vi "AlliGator Computer IRF t_0 and Mean Lifetime.vi"(8 "error in":errorcluster, 11 "Reference Decay":cluster{"t Array":dbl[], "I Array":dbl[]}) -> (0 "error out":errorcluster, 1 "t_0":dbl, 2 "<tau>_IRF":dbl)   [LabVIEW 2021, in "AlliGator Decay Processing.lvlib"]
doc: "Computes an estimate of the average lifetime of the IRF and the location of the rising time."
uses:
  AlliGator Decay Processing.lvlib
  Settings/AlliGator Settings List.ctl
  Settings/AlliGator Average Lifetime Options.ctl
  Graphs/XY Graph/XY Graph Add-Ons.lvlib
  Settings/AlliGator Settings.lvlib
  IRF/AlliGator IRF.lvlib
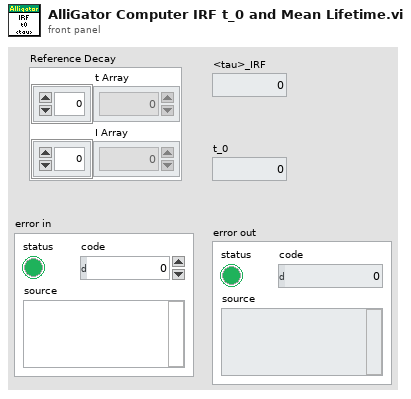
[diagram p1: front panel]
types:
  T1 = typedef "AlliGator Settings.lvlib/AlliGator Average Lifetime Options.ctl" = cluster{"Use Local IRF ":bool, "Use IRF Offset":bool, "Use Fixed Offset":bool, "Fixed Offset":dbl[unit], "Baseline %":dbl}
  T2 = typedef "AlliGator Settings.lvlib/AlliGator Settings List.ctl" = enum16{"GUI:Visible Settings Tab", "GUI:Last Run Version", "Source Image:Use Image Histogram for Contrast", "Source Image:Low Count Pixels Rejection Options", "Source Image:High Count Pixels Rejection Options", "Source Image:Use Image Brightness", "Source Image:Blend Overlay with Image Background", "Source Image:Use Fixed ROI Diameter", "Source Image:ROI Diameter", "Source Image:ROI Center Color", "Source Image:Peak Threshold", "Source Image:Intensity Threshold", "Source Image:Image Binning Options", "Source Image:Image Smoothing Options", "Source Image:Image Histogram Active", "Source Image:Invert Binary Mask", "Source Image:Hot Pixel Removal", "Source Image:Overlay Analyzed ROI Center", "Source Image:Auto-Adjust Contrast", "Source Image:Histogram Lower Percentile", "Source Image:Histogram Upper Percentile", "Source Image:Save Source Image", "Source Image:Scale Bar Options", "Source Image:Image Resolution (Pixel Size)", "Source Image:Flatfield Correction", "Source Image:Show Dead Left Columns Correction", "Source Image:Dead Left Columns Correction", "Source Image:Image Pre-Processing Operations Order", "Source Image:Overlay ROI Median", "Source Image:Median Overlay Color", "Data Information:Gate Width", "Data Information:Nanotime Gate Separation", "Data Information:Macrotime Gate Separation", "Data Information:Gate Step", "Data Information:# Gates", "Data Information:Gate Image Exposure", "Data Information:Gate Image Integration", "Data Information:Gates to Skip", "Data Information:Gates to Keep", "Data Information:Define Gates to", "Data Information:Channel Name", "Data Information:Available Channel Names", "Data Information:Channel Arithmetic", "Data Information:Background File Subtraction", "Data Information:Background File", "Data Information:Background Scaling Factor", "Data Information:Background Pile-up Correction", "Data Information:Background Pixel Well Capacity", "Data Information:Laser Period", "Data Information:SYNC Period", "Data Information:Pile-up Correction", "Data Information:Pixel Well Capacity", "Data Information:Dataset Scaling Factor", "Fluorescence Decay_Decay Pre-Processing:Reverse Gates", "Fluorescence Decay_Decay Pre-Processing:Verbose Decay Pre-Processing", "Fluorescence Decay_Decay Pre-Processing:Use Decay Pre-Processing", "Fluorescence Decay_Decay Pre-Processing:Background Subtraction", "Fluorescence Decay_Decay Pre-Processing:Background Definition Range", "Fluorescence Decay_Decay Pre-Processing:Baseline Subtraction Method", "Fluorescence Decay_Decay Pre-Processing:Decay Pre-Processing Operations Order", "Fluorescence Decay_Decay Pre-Processing:Smoothing Parameter", "Fluorescence Decay_Decay Pre-Processing:Shift Decay", "Fluorescence Decay_Decay Pre-Processing:Decay Shift Parameters", "Fluorescence Decay_Decay Pre-Processing:Fold Decay", "Fluorescence Decay_Decay Pre-Processing:# Folds", "Fluorescence Decay_Decay Pre-Processing:1-Normalize Decay", "Fluorescence Decay_Decay Pre-Processing:[0-1]-Normalize Decay", "Fluorescence Decay_Decay Pre-Processing:Smoothen Decay", "Fluorescence Decay_Decay Pre-Processing:Extrapolate Decay", "Fluorescence Decay_Decay Pre-Processing:Use Periodicity", "Fluorescence Decay_Decay Pre-Processing:Use Cursors", "Fluorescence Decay_Decay Pre-Processing:Tail Fraction", "Fluorescence Decay_Decay Pre-Processing:Head Fraction", "Fluorescence Decay_Decay Pre-Processing:Additional Points", "Fluorescence Decay_Decay Pre-Processing:Straighten Decay", "Fluorescence Decay_Decay Pre-Processing:Constant Background", "Fluorescence Decay_Decay Pre-Processing:Pixel-Normalize Decay", "Fluorescence Decay_Advanced Analysis:Extract IRF instead of Decay", "Fluorescence Decay_Advanced Analysis:IRF Extraction Options", "Fluorescence Decay_Advanced Analysis:IRF Optimization Options", "Fluorescence Decay_Advanced Analysis:Square Pulse Options", "Fluorescence Decay_Advanced Analysis:IRF Order", "Fluorescence Decay_Advanced Analysis:IRF Time Constants", "Fluorescence Decay_Advanced Analysis:Wavelet Analysis Options", "Fluorescence Decay_Advanced Analysis:Average Lifetime Options", "Fluorescence Decay_Fit Options:Fit Options", "Fluorescence Decay_Fit Options:Use Legacy Fitting Approach", "Fluorescence Decay_Fit Options:Use Data Information Laser Period", "Fluorescence Decay_Fit Parameters:Displayed Fit Parameters", "Fluorescence Decay_Fit Parameters:Fit Parameter Constraints", "Fluorescence Decay_Fit Parameters:Export Tabulated Results", "Fluorescence Decay_Fit Parameters:MLE Baseline Offset Type", "Fluorescence Decay_Fit Parameters:MLE Baseline Offset", "Fluorescence Decay_Fit Parameters:Guess Parameter Names", "Fluorescence Decay_Fit Parameters:Guess Parameter Values", "Fluorescence Decay_Fit Parameters:Guess Parameters Options", "Fluorescence Decay_Styles:Show Last Decay Only", "Fluorescence Decay_Styles:Decay Graph Color Array", "Fluorescence Decay:Decay Graph Active", "Fluorescence Decay Statistics:Min Peak Value", "Fluorescence Decay Statistics:Reject Low Decay Peak Pixels", "Fluorescence Decay Statistics:Reject High Decay Peak Pixels", "Fluorescence Decay Statistics:Max Peak Value", "Time Traces:Use File Timestamp", "Time Traces:Time Step", "Time Traces:Use Intensity Correction File", "Time Traces:Intensity Correction File", "Phasor Plot:Phasor Plot Smoothing Options", "Phasor Plot:Phasor Plot Size", "Phasor Plot:Phasor Plot Graphics Options", "Phasor Plot:Cumulative Phasor Plot", "Phasor Plot:Use Phasor Brightness", "Phasor Plot:Blend Overlay with Phasor Background", "Phasor Plot:Save Phasor Plot", "Phasor Plot:Show References", "Phasor Plot:Phasor Ratio Decay Range", "Phasor Plot:Exponential Fading", "Phasor Plot:Phasor Ratio Reference Colors", "Phasor Plot:Reference Radius", "Phasor Plot:Show Color Map Vertices", "Phasor Plot:Phasor Plot Active", "Phasor Plot:Phasor Ratio Color Map Type", "Phasor Plot:Phasor Ratio Color Map", "Phasor Plot:Phasor Ratio Display Range", "Phasor Plot:Selected Image ROI(s)", "Phasor Plot:All Image ROIs", "Phasor Plot:Selected Phasor Plot ROI(s)", "Phasor Plot:All Phasor Plot ROIs", "Phasor Plot:Phasor Ratio Color-Coded Quantity", "Phasor Plot:Store Phasor Harmonics", "Phasor Plot:Draw Reference Segment", "Phasor Plot:User-Defined Quantity", "Phasor Graph:Phasor Frequency", "Phasor Graph:Phasor Ratio Type", "Phasor Graph:Pixel-level Phasor Computation", "Phasor Graph:Save Phasor Graph", "Phasor Graph:Phasor Graph Active", "Phasor Graph:Phasor SDV Options", "Phasor Calibration:Use Backup Calibration if needed", "Phasor Graph:Define Shortest Lifetime as", "Phasor Calibration:Backup Calibration Type", "Phasor Calibration:Calibration Type", "Phasor Calibration:Calibration Lifetime", "Phasor Calibration:Calibration Map Algorithm", "Single-Exponential Phasor Locus (SEPL):Gate Parameters", "Single-Exponential Phasor Locus (SEPL):User-defined Gate", "Single-Exponential Phasor Locus (SEPL):User-defined IRF", "Single-Exponential Phasor Locus (SEPL):Phasor Parameters", "Single-Exponential Phasor Locus (SEPL):Decay & IRF Parameters", "Single-Exponential Phasor Locus (SEPL):Display Parameters", "Lifetime Analysis:Decay Analysis Parameters", "Lifetime Analysis:Lifetime Map Active", "Plugins:Python Settings", "Miscellaneous:Verbose Mode", "Miscellaneous:Beep after Script", "Miscellaneous:Saved Image File Format", "Miscellaneous:Exported Gate Image Settings", "Miscellaneous:Include Loading in Timing", "Miscellaneous:Verbose Settings Mode", "Miscellaneous:Histogram Options", "Miscellaneous:Beep on Error", "Miscellaneous:# Logical Processors Used", "Miscellaneous:ROI Description Max Characters", "Miscellaneous:Verbose Error Mode", "Miscellaneous:Transparent Mask Color"}
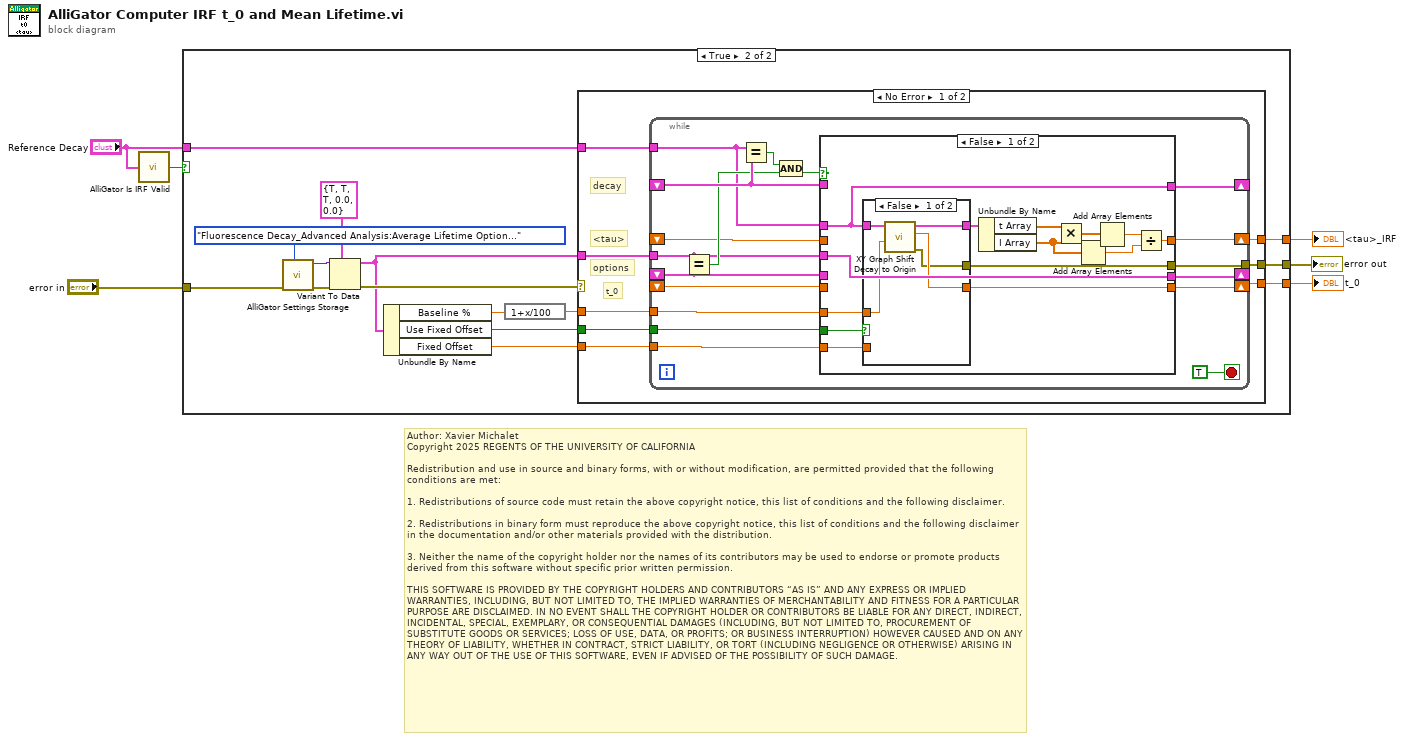
[diagram p0: block diagram]
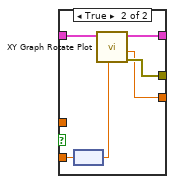
[diagram p3: hidden frame]
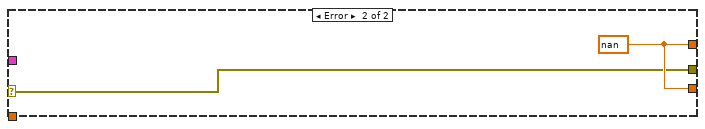
[diagram p5: hidden frame]
diagram:
  # "Author: Xavier Michalet\nCopyright 2025 REGENTS OF THE UNIVERSITY OF CALIFORNIA\n\nRedistribution and use in source and binary forms, with or without modification, are permitted provided that the following conditions are met:\n\n1. Redistributions of source code must retain the above copyright notice, this list of conditions and the following disclaimer.\n\n2. Redistributions in binary form must reproduce the above copyright notice, this list of conditions and the following disclaimer in the documentation and/or other materials provided with the distribution.\n\n3. Neither the name of the copyright holder nor the names of its contributors may be used to endorse or promote products derived from this software without specific prior written permission.\n\nTHIS SOFTWARE IS PROVIDED BY THE COPYRIGHT HOLDERS AND CONTRIBUTORS “AS IS” AND ANY EXPRESS OR IMPLIED WARRANTIES, INCLUDING, BUT NOT LIMITED TO, THE IMPLIED WARRANTIES OF MERCHANTABILITY AND FITNESS FOR A PARTICULAR PURPOSE ARE DISCLAIMED. IN NO EVENT SHALL THE COPYRIGHT HOLDER OR CONTRIBUTORS BE LIABLE FOR ANY DIRECT, INDIRECT, INCIDENTAL, SPECIAL, EXEMPLARY, OR CONSEQUENTIAL DAMAGES (INCLUDING, BUT NOT LIMITED TO, PROCUREMENT OF SUBSTITUTE GOODS OR SERVICES; LOSS OF USE, DATA, OR PROFITS; OR BUSINESS INTERRUPTION) HOWEVER CAUSED AND ON ANY THEORY OF LIABILITY, WHETHER IN CONTRACT, STRICT LIABILITY, OR TORT (INCLUDING NEGLIGENCE OR OTHERWISE) ARISING IN ANY WAY OUT OF THE USE OF THIS SOFTWARE, EVEN IF ADVISED OF THE POSSIBILITY OF SUCH DAMAGE."
  n1 = call "AlliGator Is IRF Valid.vi"("Reference Decay"="Reference Decay") -> ("Valid Plot?"=w1:bool)  [unwired: 8 in]
  n2 = case shown="True" w1 {
    tunnel: [_ w22] -> w6
    tunnel: [w7 w21] -> w5
    tunnel: [_ w20] -> w4
    tunnel: "error in" -> [w7 w15]
    tunnel: "Reference Decay" -> [_ w8]
    frame False {
      # "invalid IRF: ignore."
    }
    frame True {
      n3 = call "AlliGator Settings Storage.vi"("AlliGator Settings List"=AlliGator_Settings_List."Fluorescence Decay_Advanced Analysis:Average Lifetime Options", "Error In"=w15) -> ("Error Out"=w16:errorcluster, "Variant Data out"=w18:variant)  [unwired: 8 in]
      n4 = Variant To Data(error in=w16, type=T1 {"Use Local IRF "=TRUE, "Use IRF Offset"=TRUE, "Use Fixed Offset"=TRUE, "Fixed Offset"=0.0, "Baseline %"=0.0} ("Average Lifetime Options"), Variant=w18) -> (data=w11:T1, error out=w14:errorcluster)
      n5 = Unbundle By Name(w11) -> ("Baseline %"=w13:dbl, "Use Fixed Offset"=w10:bool, "Fixed Offset"=w9:dbl[unit])
      n6 = expression code="1+x/100"(w13) -> (w12:dbl)
      n7 = case shown="No Error" w14 {
        selector: w14 -> [_ w78]
        tunnel: [w30 w79] -> w22
        tunnel: [w29 w78] -> w21
        tunnel: [w28 w79] -> w20
        tunnel: w12 -> [w27 _]
        tunnel: w11 -> [w26 _]
        tunnel: w10 -> [w25 _]
        tunnel: w9 -> [w24 _]
        tunnel: w8 -> [w23 _]
        frame No Error {
          # "t_0"
          # "options"
          # "<tau>"
          # "decay"
          n8 = while {
            tunnel: [w44] -> w29
            shift-right: [w46] -> _
            shift-left: _ -> [w47]
            shift-right: [w45] -> w28
            shift-left: _ -> [w34]
            shift-right: [w42] -> w30
            shift-left: _ -> [w41]
            tunnel: w27 -> [w39]
            tunnel: w26 -> [w35]
            shift-right: [w43] -> _
            shift-left: _ -> [w36]
            tunnel: w25 -> [w38]
            tunnel: w24 -> [w37]
            tunnel: w23 -> [w32]
            stop <- TRUE stop-if-true
            n9 = Equal?(x=w35, y=w36) -> (x = y?=w40:bool)
            n10 = Equal?(x=w32, y=w47) -> (x = y?=w31:bool)
            n11 = Compound Arithmetic op=AND(w31, w40) -> (w33:bool)
            n12 = case shown="False" w33 {
              tunnel: [w61 w76] -> w42
              tunnel: w32 -> [w49 _]
              tunnel: [w55 w77] -> w45
              tunnel: [w49 w74] -> w46
              tunnel: w47 -> [_ w74]
              tunnel: w34 -> [_ w77]
              tunnel: w41 -> [_ w76]
              tunnel: [w54 _] -> w44
              tunnel: w39 -> [w53 _]
              tunnel: w36 -> [_ w75]
              tunnel: [w52 w75] -> w43
              tunnel: w35 -> [w52 _]
              tunnel: w38 -> [w51 _]
              tunnel: w37 -> [w50 _]
              frame False {
                n13 = case shown="False" w51 {
                  tunnel: [w67 w72] -> w62
                  tunnel: [w66 w70] -> w61
                  tunnel: w49 -> [w65 w73]
                  tunnel: [w64 w71] -> w54
                  tunnel: w53 -> [w63 _]
                  tunnel: w50 -> [_ w69]
                  frame False {
                    n14 = call "XY Graph Shift Decay to Origin.vi"("tolerance factor (1.2)"=w63, "Decay in"=w65) -> ("error out"=w64:errorcluster, "t_0"=w66:dbl, "Rotated Decay out"=w67:cluster{"t Array":dbl[], "I Array":dbl[]})  [unwired: 6 in, 1 out]
                  }
                  frame True {
                    n15 = node(w69) -> (w68:dbl)
                    n16 = call "XY Graph Rotate Plot.vi"("t_0 (NaN: use index)"=w68, "Decay in"=w73) -> ("Error Out"=w71:errorcluster, "t_0"=w70:dbl, "Decay out"=w72:cluster{"t Array":dbl[], "I Array":dbl[]})  [unwired: 7 in]
                  }
                }
                n17 = Unbundle By Name(w62) -> ("t Array"=w57:dbl[], "I Array"=w56:dbl[])
                n18 = Multiply(x=w57, y=w56) -> (x*y=w58:dbl[])
                n19 = Add Array Elements(numeric array=w56) -> (sum=w60:dbl)
                n20 = Add Array Elements(numeric array=w58) -> (sum=w59:dbl)
                n21 = Divide(x=w59, y=w60) -> (x/y=w55:dbl)
              }
              frame True {
                # "use previous values"
              }
            }
          }
        }
        frame Error {
          w79 = nan
        }
      }
    }
  }
  "t_0" <- w6
  "<tau>_IRF" <- w4
  "error out" <- w5
